vi "MoveAcquiredData (SubVI).vi"(7 "Bytes/Readout >":i32, 8 "error in (no error)":errorcluster, 9 "readout_count":i64, 10 "initial_readout*":u64, 11 "DataAcquisitionBuffer in":T1) -> (0 "error out":errorcluster, 3 "DataAcquisitionBuffer out":T1)   [LabVIEW 2019, in "PICam.lvlib"]
uses:
  PICam.lvlib
  types/utility/DataAcquisitionResult.ctl
  types/PicamRoi.ctl
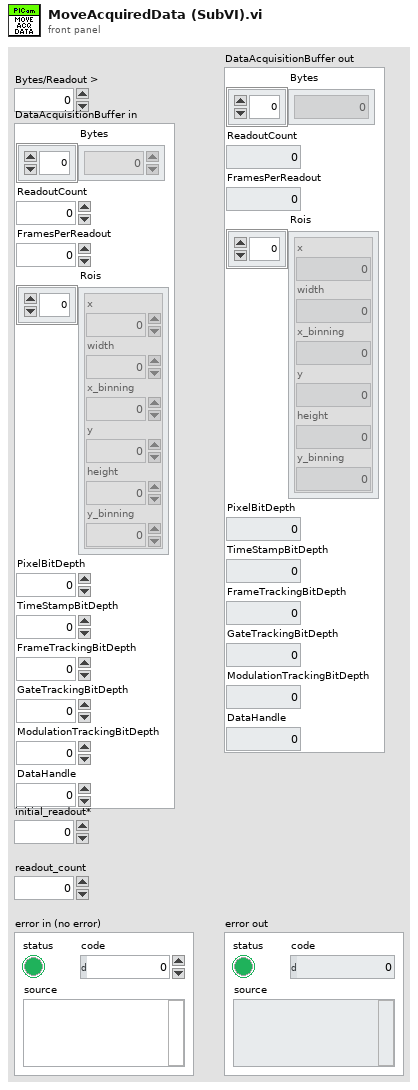
[diagram p1: front panel]
types:
  T1 = typedef "PICam.lvlib/DataAcquisitionResult.ctl" = cluster{"Bytes":u8[], "ReadoutCount":i64, "FramesPerReadout":i32, "Rois":T2[], "PixelBitDepth":i32, "TimeStampBitDepth":i32, "FrameTrackingBitDepth":i32, "GateTrackingBitDepth":i32, "ModulationTrackingBitDepth":i32, "DataHandle":u64}
  T2 = typedef "PicamRoi.ctl" = cluster{"x":i32, "width":i32, "x_binning":i32, "y":i32, "height":i32, "y_binning":i32}
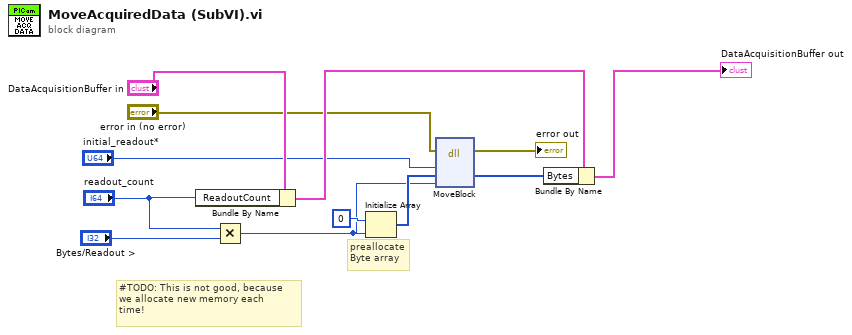
[diagram p0: block diagram]
diagram:
  # "#TODO: This is not good, because\nwe allocate new memory each\ntime!"
  # "preallocate\nByte array"
  n1 = Bundle By Name(cluster="DataAcquisitionBuffer in", "ReadoutCount"="readout_count") -> (w9:T1)
  n2 = Multiply(x="readout_count", y="Bytes/Readout >") -> (x*y=w1:i64)
  n3 = Initialize Array(u8 0 ("element"), w1) -> (w5:u8[])
  n4 = dll-call lib="LabVIEW" fn="MoveBlock"(error in="error in (no error)", "src"="initial_readout*", "dest"=w5, "size"=w1) -> (error out=→"error out":errorcluster, "dest"=w11:u8[])  [unwired: 5 in, 1 out]
  n5 = Bundle By Name(cluster=w9, "Bytes"=w11) -> (→"DataAcquisitionBuffer out":T1)
